vi "LIA7230_read_sens.vi"(8 "error in (no error)":errorcluster, 10 "Reference Mode":bool, 11 "VISA session (in)":refnum<visa-resource-name>) -> (0 "error out":errorcluster, 2 "Range Out":u8 step=1, 3 "VISA session (out)":refnum<visa-resource-name>)   [LabVIEW 2019]
uses:
  Equipment/LIA7230/SR7230LV8.llb/SR7230 VISA Write/Read.vi
panel:
  # "Dual"
  # "Single"
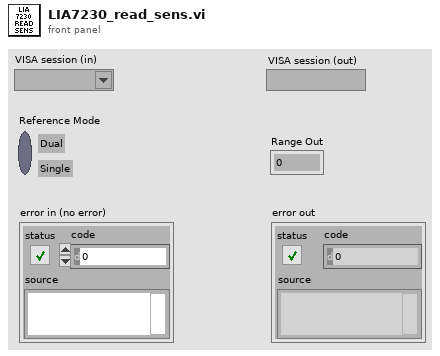
[diagram p1: front panel]
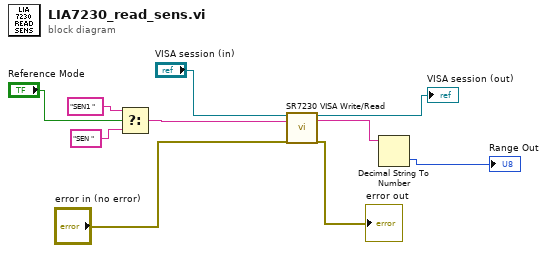
[diagram p0: block diagram]
diagram:
  n1 = Select(t="SEN1 ", s="Reference Mode", f="SEN ") -> (s? t:f=w7:string)
  n2 = call "SR7230 VISA Write/Read.vi"("VISA session (for class)"="VISA session (in)", "Write Command String"=w7, "error in (no error)"="error in (no error)") -> ("VISA session"=→"VISA session (out)":refnum<visa-resource-name>, "Response 1"=w4:string, "error out"=→"error out":errorcluster)  [unwired: 4 in, 10 out]
  n3 = Decimal String To Number(string=w4) -> (number=→"Range Out":i32)  [unwired: 2 in, 1 out]
